vi "Close All Comm Connections.vi"(7 "Name":string, 8 "error in":errorcluster, 10 "ref in":T1, 11 "listener ID":refnum<k5>) -> (0 "error out":errorcluster)   [LabVIEW 2015, in "Diagnostics Addon Engine.lvlib"]
uses:
  <vilib>/NI/STM/Connection Manager/TCP/Advanced/TCP Connection Manager Reference.ctl
  <vilib>/NI/STM/Connection Manager/TCP/Advanced/TCP Connection Manager State Variables.ctl
  <vilib>/NI/STM/TCP/TCP Connection Info.ctl
  <vilib>/NI/STM/SubVIs/MetaDataElement.ctl
  <vilib>/NI/STM/Connection Manager/TCP/TCP Connection Properties.ctl
  <vilib>/NI/STM/Connection Manager/TCP/TCP Connection Method.ctl
  Diagnostics Addon Engine.lvlib
  <vilib>/NI Veristand/Custom Device Tools/Custom Device Utility Library/Custom Device Utility Library.lvlib
  <vilib>/NI/STM/NI STM.lvlib
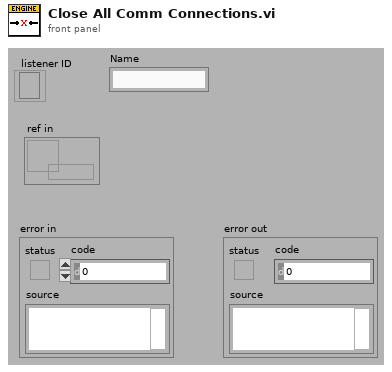
[diagram p1: front panel]
types:
  T1 = typedef "TCP Connection Manager Reference.ctl" = refnum<data-value>
  T2 = typedef "NI STM.lvlib/TCP Connection Method.ctl" = enum16{"Initialize", "Add Connection", "Set Properties", "Get Connection(s)", "Remove Connection", "Remove All Connections", "Get Connection Count"}
  T3 = typedef "NI STM.lvlib/TCP Connection Info.ctl" = cluster{"connection ID":refnum<k5>, "meta data":T4[]}
  T4 = typedef "NI STM.lvlib/MetaDataElement.ctl" = string
  T5 = typedef "NI STM.lvlib/TCP Connection Properties.ctl" = cluster{"Name":string, "Address":string, "Custom":string}
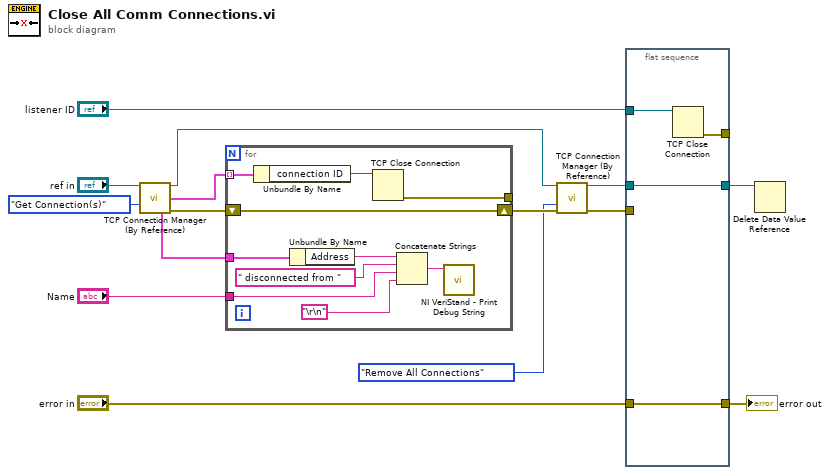
[diagram p0: block diagram]
diagram:
  n1 = call <vilib>:"TCP Connection Manager (By Reference).vi"("connection manager ref in"="ref in", "method"=TCP_Connection_Method."Get Connection(s)") -> ("connection manager ref out"=w5:T1, "all connections"=w12:T3[], "properties out"=w3:T5, "error out"=w11:errorcluster)  [unwired: 7 in, 3 out]
  n2 = for {
    tunnel: w12 -> [w17] mode=indexing
    shift-right: [w23] -> w10
    shift-left: w11 -> [w23]
    tunnel: [w24] -> _
    tunnel: "Name" -> [w19]
    tunnel: w3 -> [w18]
    n3 = Unbundle By Name(w17) -> ("connection ID"=w25:refnum<k5>)
    n4 = Unbundle By Name(w18) -> ("Address"=w20:string)
    n5 = TCP Close Connection(connection ID=w25) -> (error out=w24:errorcluster)  [unwired: 2 in, 1 out]
    n6 = Concatenate Strings(w20, " disconnected from " ("string"), w19, "\r\n") -> (w22:string)
    n7 = call <vilib>:"NI VeriStand - Print Debug String.vi"("Message"=w22) -> ()  [unwired: 10 in, 1 out]
  }
  n8 = call <vilib>:"TCP Connection Manager (By Reference).vi"("connection manager ref in"=w5, "method"=TCP_Connection_Method."Remove All Connections", "error in"=w10) -> ("connection manager ref out"=w7:T1, "error out"=w9:errorcluster)  [unwired: 6 in, 5 out]
  n9 = flat-sequence {
    tunnel: "listener ID" -> [w29]
    tunnel: [w28] -> w14
    tunnel: w9 -> [_]
    tunnel: "error in" -> [w28]
    tunnel: [w27] -> _
    tunnel: w7 -> [w26]
    tunnel: [w26] -> w6
    frame #0 {
      n10 = TCP Close Connection(connection ID=w29) -> (error out=w27:errorcluster)  [unwired: 2 in, 1 out]
    }
  }
  n11 = Delete Data Value Reference(data value reference=w6) -> ()  [unwired: 1 in, 2 out]
  "error out" <- w14
